vi "sendEnterKey.vi"   [LabVIEW 2021]
doc: "This is an example that shows how to have a message box pop up and exit with out having to press OK."
uses:
  user32.dll
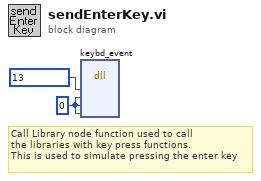
[diagram p0: block diagram]
diagram:
  w1 = u8 0 ("bScan")
  # "Call Library node function used to call \nthe libraries with key press functions. \nThis is used to simulate pressing the enter key"
  n1 = dll-call lib="user32.dll" fn="keybd_event"("bVk"=u8 13 ("Virtual Key"), "bScan"=w1, "dwFlags"=w1, "dwExtraInfo"=w1) -> ()  [unwired: 8 in, 2 out]
